vi "TDC_switchTermination.vi"(8 "Error In":errorcluster, 11 "Input Termination":bool) -> (0 "Error Out":errorcluster)   [LabVIEW 2011]
uses:
  dist/userlib/lib/tdcbase.dll
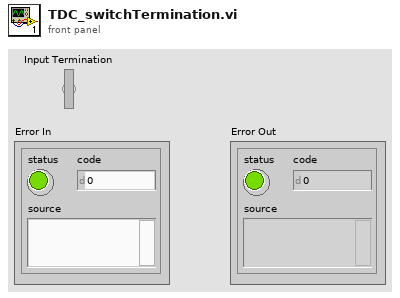
[diagram p1: front panel]
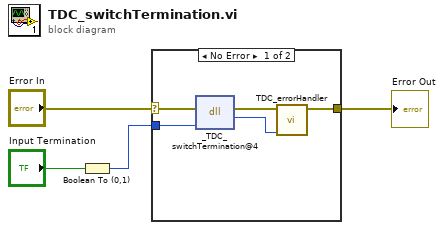
[diagram p0: block diagram]
diagram:
  n1 = Boolean To (0,1)(Boolean="Input Termination") -> (0, 1=w1:i16)
  n2 = case shown="No Error" "Error In" {
    selector: "Error In" -> [w8 w10]
    tunnel: [w6 w10] -> w3
    tunnel: w1 -> [w9 _]
    frame No Error {
      n3 = dll-call lib="C:/nh/projekt/spmctrl/dist/userlib/lib/tdcbase.dll" fn="_TDC_switchTermination@4"(error in=w8, "on"=w9) -> (error out=w7:errorcluster, "return type"=w5:i32)  [unwired: 3 in, 1 out]
      n4 = call "TDC_errorHandler.vi"("quTAU Return Code"=w5, "Error In"=w7) -> ("Error Out"=w6:errorcluster)  [unwired: 9 in]
    }
    frame Error {
    }
  }
  "Error Out" <- w3
